vi "HAPS_LoadTable_Manual_Selected_Any_Preamp.vi"() -> ()   [LabVIEW 2023, in "HAPS.lvlib"]
uses:
  HAPS.lvlib
  set_ele.ctl
  HAPS_SerialPort.ctl
  HAPS_MCU_ELE_Func.ctl
  <vilib>/Utility/file.llb/Read Delimited Spreadsheet (string).vi
  R_S/R_S.lvlib
panel:
  in  "file path":path=path "D:/_Project/_Code/LabVIEW/_CLC_Gen4/CLC_LV2023/CLC_Cali/Log/HAPS/Preset.csv"
  in  "Preamp_Channel":bool[](array[boolean])
  in  "offset":i32=16
  in  "H_V?":bool
  in  "IC_On/OFF":bool[][](array[boolean])=[[FALSE, FALSE, FALSE, FALSE, FALSE, FALSE, FALSE, FALSE, FALSE, FALSE, FALSE, FALSE], [FALSE, FALSE, FALSE, FALSE, FALSE, FALSE, FALSE, FALSE, FALSE, FALSE, FALSE, FALSE], [FALSE, FALSE, FALSE, FALSE, FALSE, FALSE, FALSE, FALSE, FALSE, FALSE, FALSE, FALSE]]
  in  "ele_gain?":i32=35
  in  "sys reboot?":bool=TRUE
  in  "VISA resource name":refnum<visa-resource-name>="COM1"
  out "error IO":errorcluster
  out "Err_code":i32
  out "status":bool
  in  "offset?":bool
  in  "simu.?":bool
  in  "set_ele":T1={"ch"=0, "chain_id"=0, "group"=0, "array_id"=0, "ele_phase"=0, "ele_gain"=35, "com_gain"=17, "pd_range"=0}
  out "ele phase":i32
  out "ele gain":i32
  out "channel":i32
  out "chain ID":i32
  out "group":i32
  out "array id":i32
  # "HAPS 24x24 Setting Manual In-Phase : \n                                              Any BFIC & Preamp"
  # "Tx:35\nRx:22"
  # "0"
  # "5"
  # "6"
  # "11"
  # "Group_0"
  # "Group_1"
  # "Group_2"
  # "Not using!!!!!!!!!!!!!!!!!!!!!!!!!!!!!!!!!!!!!!!!"
  # "0        1       2        3        4       5        6       7        8        9      10      11     12     13     14      15"
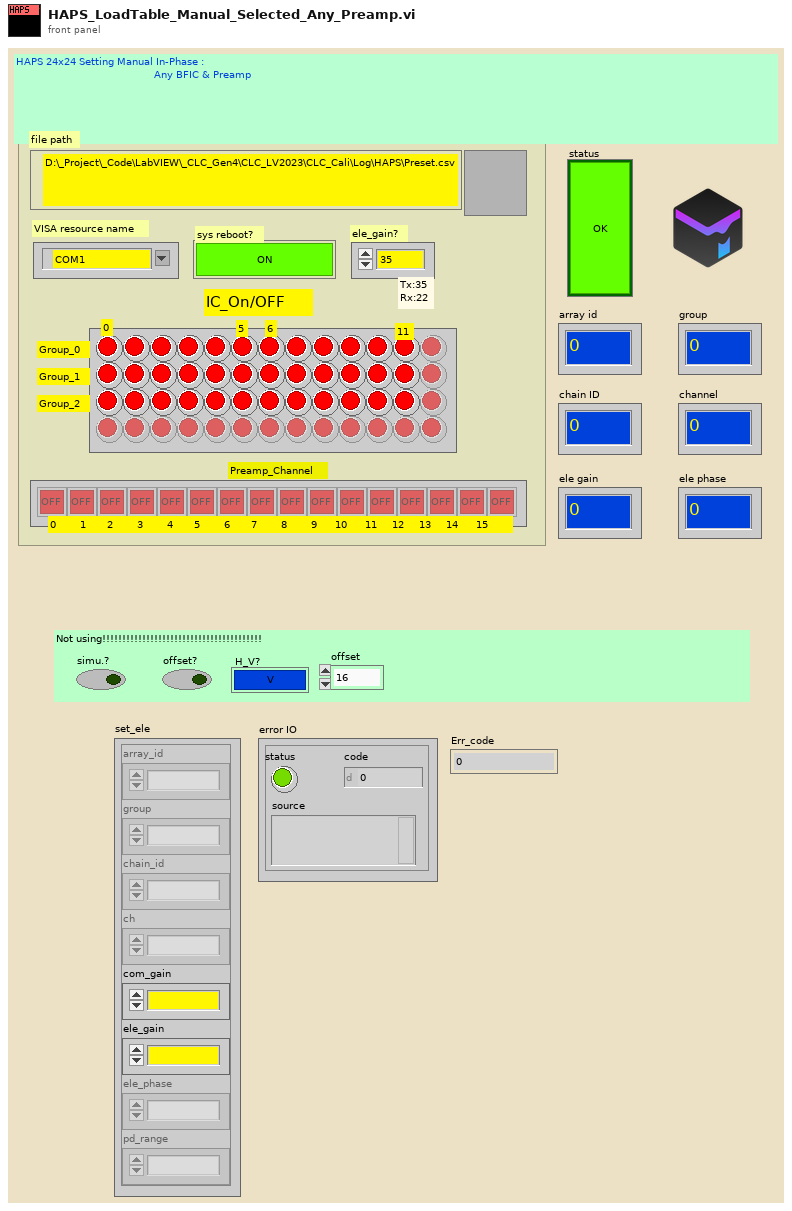
[diagram p1: front panel]
types:
  T1 = typedef "HAPS.lvlib/set_ele.ctl" = cluster{"ch":i32, "chain_id":i32, "group":i32, "array_id":i32, "ele_phase":i32, "ele_gain":i32, "com_gain":i32, "pd_range":i32}
  T2 = typedef "HAPS.lvlib/HAPS_SerialPort.ctl" = enum16{"Init", "Close", "CMD", "Flush"}
  T3 = typedef "HAPS.lvlib/HAPS_MCU_ELE_Func.ctl" = enum16{"array_init", "set_com_gain", "set_ch_gain_phase", "set_pd_range", "get_preamp_temp", "get_bfic_temp", "get_tx_pd", "ch_on", "ch_on_2", "ch_ctrl_all", "array_ctrl_src"}
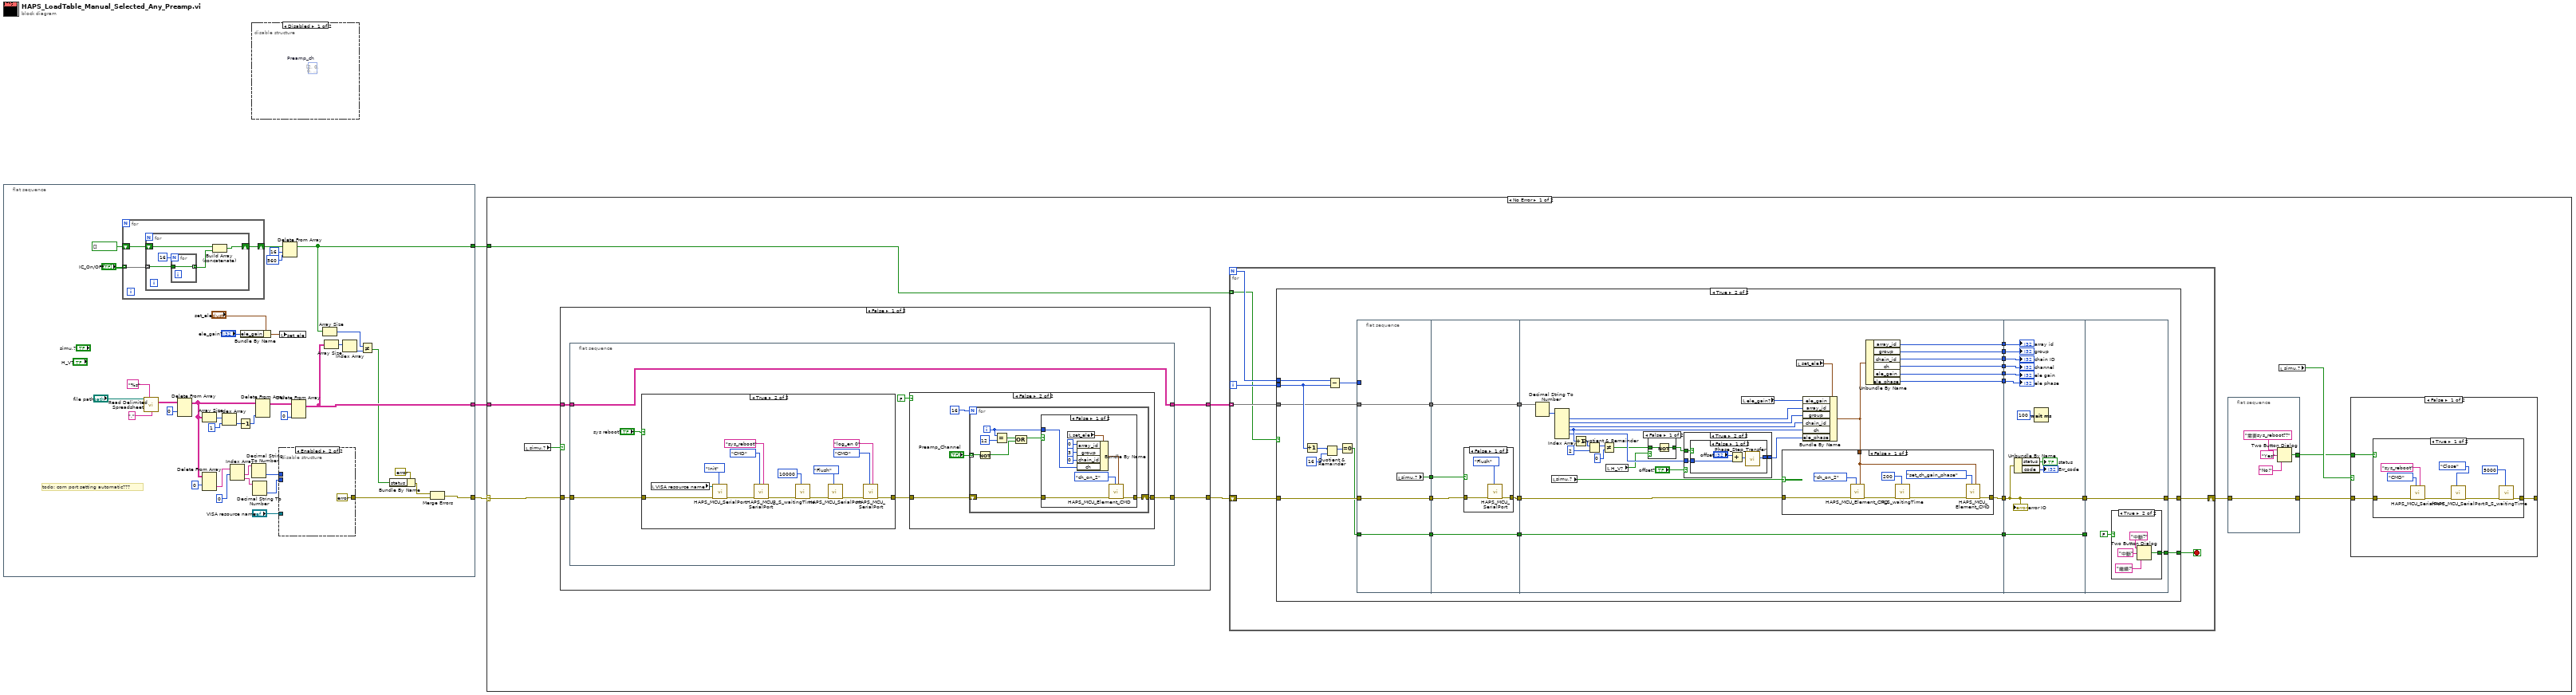
[diagram p0: block diagram]
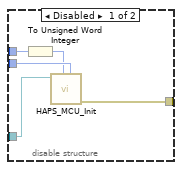
[diagram p2: hidden frame]
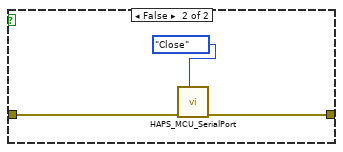
[diagram p4: hidden frame]
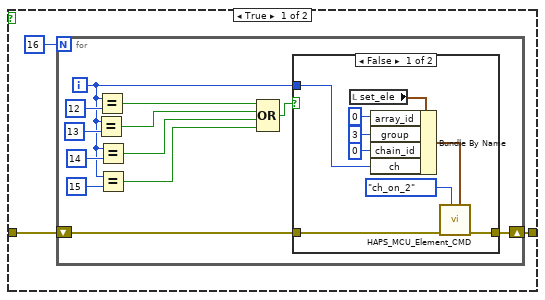
[diagram p6: hidden frame]
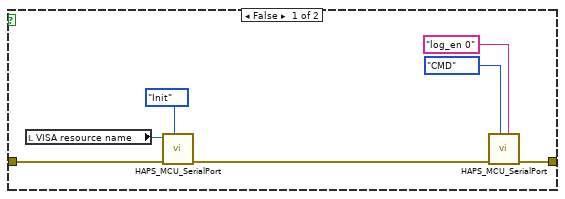
[diagram p9: hidden frame]
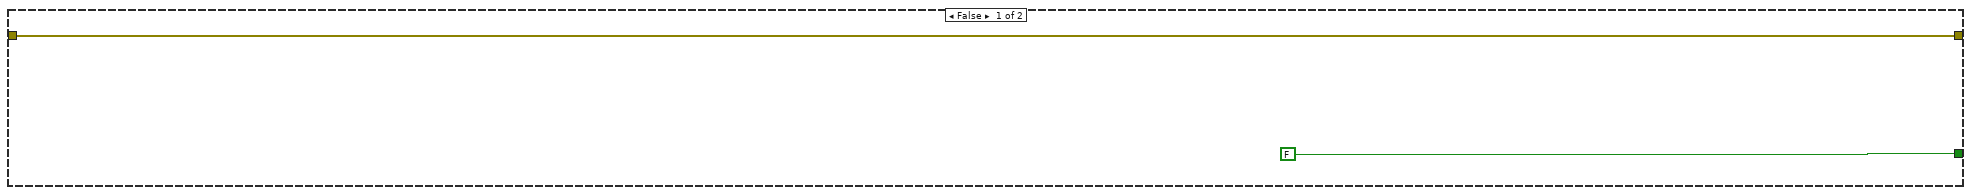
[diagram p11: hidden frame]
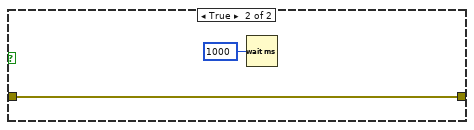
[diagram p16: hidden frame]
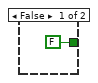
[diagram p17: hidden frame]
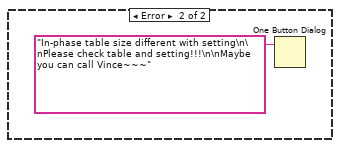
[diagram p18: hidden frame]
diagram:
  n1 = flat-sequence {
    tunnel: [w7] -> w3
    tunnel: [w11] -> w2
    tunnel: [w12] -> w1
    frame #0 {
      # "todo: com port setting automatic???"
      n2 = for {
        tunnel: "IC_On/OFF" -> [w44] mode=indexing
        shift-right: [w42] -> w17
        shift-left: bool[] [] -> [w43]
        n3 = for {
          tunnel: w44 -> [w48] mode=indexing
          shift-right: [w45] -> w42
          shift-left: w43 -> [w46]
          n4 = for {
            N: 16 -> [_]
            tunnel: w48 -> [w50]
            tunnel: [w50] -> w47 mode=indexing
          }
          n5 = Build Array (concatenate)(w46, w47) -> (w45:bool[])
        }
      }
      n6 = call-poly <vilib>:"Read Delimited Spreadsheet.vi"("file path (dialog if empty)"="file path", "format (%s)"="%s" ("format (%.3f)"), "delimiter (\\t)"="," ("delimiter (\\t)")) -> ("all rows"=w39:string[][])  [unwired: 7 in, 5 out]
      n7 = Delete From Array(array=w39, index (row)=0) -> (array with subset deleted=w29:string[][])  [unwired: 2 in, 1 out]
      n8 = Array Size(array=w29) -> (size(s)=w37:i32[])
      n9 = Delete From Array(array=w29, index (row)=0) -> (deleted portion=w28:string[])  [unwired: 2 in, 1 out]
      n10 = Index Array(array=w37, index=1) -> (element=w34:i32)
      n11 = Index Array(array=w28, index #1=0 ("index")) -> (element #1=w27:string, element #2=w26:string)  [unwired: 1 in]
      n12 = Decrement(x=w34) -> (x-1=w36:i32)
      n13 = Bundle By Name(cluster="set_ele", "ele_gain"="ele_gain?") -> (w18:T1)
      n14 = Decimal String To Number(string=w27) -> (number=w23:i32)  [unwired: 2 in, 1 out]
      n15 = Decimal String To Number(string=w26) -> (number=w22:i32)  [unwired: 2 in, 1 out]
      n16 = Delete From Array(array=w29, index (col)=w36) -> (array with subset deleted=w32:string[][])  [unwired: 2 in, 1 out]
      n17 = disable-structure shown="Enabled" {
        disable-tunnel: [w55 errorcluster {"status"=FALSE, "code"=0, "source"=""} ("error out")] -> w33
        disable-tunnel: w23 -> [w54 _]
        disable-tunnel: w22 -> [w53 _]
        disable-tunnel: "VISA resource name" -> [w52 _]
        frame Disabled {
          n18 = To Unsigned Word Integer(number=w54) -> (unsigned 16bit integer=w51:u16)
          n19 = call "HAPS_MCU_Init.vi"("array_id"=w53, "Tx/Rx"=w51, "VISA resource name"=w52) -> ("error out"=w55:errorcluster)  [unwired: 8 in]
        }
        frame Enabled {
        }
      }
      n20 = local write "set_ele"(w18) -> ()
      n21 = Delete From Array(array=w17, length=16, index=560) -> (array with subset deleted=w12:bool[])  [unwired: 1 out]
      n22 = Delete From Array(array=w32, index (col)=0 ("index (row)")) -> (array with subset deleted=w11:string[][])  [unwired: 2 in, 1 out]
      n23 = Array Size(array=w12) -> (size(s)=w9:i32)
      n24 = Array Size(array=w11) -> (size(s)=w10:i32[])
      n25 = Index Array(array=w10) -> (element=w8:i32)  [unwired: 1 in]
      n26 = Not Equal?(x=w9, y=w8) -> (x != y?=w5:bool)
      n27 = Bundle By Name(cluster=errorcluster {"status"=FALSE, "code"=0, "source"=""} ("error out"), "status"=w5) -> (w4:errorcluster)
      n28 = Merge Errors(w4, w33) -> (w7:errorcluster)
    }
  }
  n29 = disable-structure shown="Disabled" {
    frame Disabled {
      (unwired) i32[][] [[2, 0, 0, 8, 8, 10, 11, 9, 9, 1, 1, 3], [3, 1, 1, 9, 9, 11, 13, 15, 15, 7, 7, 5], [5, 7, 7, 15, 15, 13, 14, 14, 6, 6, 4, 12]]  # Preamp_ch
    }
    frame Enabled {
    }
  }
  n30 = case shown="No Error" w3 {
    selector: w3 -> [w64 _]
    tunnel: w2 -> [w66 _]
    tunnel: w1 -> [w60 _]
    frame No Error {
      n31 = local read "simu.?"() -> (w62:bool)
      n32 = case shown="False" w62 {
        tunnel: w66 -> [w90 w166]
        tunnel: [w89 w166] -> w65
        tunnel: w64 -> [w88 w165]
        tunnel: [w87 w165] -> w63
        frame False {
          n33 = flat-sequence {
            tunnel: w90 -> [w96]
            tunnel: [w96] -> w89
            tunnel: w88 -> [w94]
            tunnel: [w95] -> w87
            frame #0 {
              n34 = case shown="True" "sys reboot?" {
                tunnel: w94 -> [w148 w162]
                tunnel: [w146 w160] -> w93
                frame False {
                  n35 = local read "VISA resource name"() -> (w144:refnum<visa-resource-name>)
                  n36 = call "HAPS_MCU_SerialPort.vi"("HAPS_SerialPort_Func"=HAPS_SerialPort."Init", "error in"=w148, "VISA resource name"=w144) -> ("error out"=w145:errorcluster)  [unwired: 6 in, 2 out]
                  n37 = call "HAPS_MCU_SerialPort.vi"("Command"="log_en 0", "HAPS_SerialPort_Func"=enum16{"Init", "Close", "CMD"}."CMD" ("HAPS_SerialPort"), "error in"=w145) -> ("error out"=w146:errorcluster)  [unwired: 6 in, 2 out]
                }
                frame True {
                  n38 = local read "VISA resource name"() -> (w151:refnum<visa-resource-name>)
                  n39 = call "HAPS_MCU_SerialPort.vi"("HAPS_SerialPort_Func"=HAPS_SerialPort."Init", "error in"=w162, "VISA resource name"=w151) -> ("error out"=w157:errorcluster)  [unwired: 6 in, 2 out]
                  n40 = call "HAPS_MCU_SerialPort.vi"("Command"="sys_reboot", "HAPS_SerialPort_Func"=enum16{"Init", "Close", "CMD"}."CMD" ("HAPS_SerialPort"), "error in"=w157) -> ("error out"=w156:errorcluster)  [unwired: 6 in, 2 out]
                  n41 = call "R_S_waitingTime.vi"("Waiting Time(ms)"=u32 10000, "error in"=w156) -> ("error out"=w154:errorcluster)  [unwired: 9 in]
                  n42 = call "HAPS_MCU_SerialPort.vi"("HAPS_SerialPort_Func"=HAPS_SerialPort."Flush", "error in"=w154) -> ("error out"=w152:errorcluster)  [unwired: 7 in, 2 out]
                  n43 = call "HAPS_MCU_SerialPort.vi"("Command"="log_en 0", "HAPS_SerialPort_Func"=enum16{"Init", "Close", "CMD"}."CMD" ("HAPS_SerialPort"), "error in"=w152) -> ("error out"=w160:errorcluster)  [unwired: 6 in, 2 out]
                }
              }
              n44 = case shown="False" FALSE {
                tunnel: [w98 w124] -> w95
                tunnel: w93 -> [w97 w123]
                frame True {
                  n45 = for {
                    N: 16 -> [_]
                    shift-right: [w110] -> w98
                    shift-left: w97 -> [w111]
                    i -> [w101]
                    n46 = Equal?(x=w101, y=13) -> (x = y?=w105:bool)
                    n47 = Equal?(x=w101, y=12) -> (x = y?=w109:bool)
                    n48 = Equal?(x=w101, y=14) -> (x = y?=w103:bool)
                    n49 = Equal?(x=w101, y=15) -> (x = y?=w100:bool)
                    n50 = Compound Arithmetic op=OR(w109, w105, w103, w100) -> (w106:bool)
                    n51 = case shown="False" w106 {
                      tunnel: w111 -> [w114 w121]
                      tunnel: [w113 w121] -> w110
                      tunnel: w101 -> [w112 _]
                      frame False {
                        n52 = local read "set_ele"() -> (w116:T1)
                        n53 = Bundle By Name(cluster=w116, "array_id"=0, "group"=3, "chain_id"=0, "ch"=w112) -> (w117:T1)
                        n54 = call "HAPS_MCU_Element_CMD.vi"("set_ele"=w117, "HAPS_MCU_ELE_Func."=HAPS_MCU_ELE_Func."ch_on_2", "error in"=w114) -> ("error out"=w113:errorcluster)  [unwired: 7 in, 1 out]
                      }
                      frame True {
                      }
                    }
                  }
                }
                frame False {
                  n55 = for {
                    N: 16 -> [_]
                    shift-right: [w132] -> w124
                    shift-left: w123 -> [w133]
                    tunnel: "Preamp_Channel" -> [w127] mode=indexing
                    i -> [w130]
                    n56 = Not(x=w127) -> (.not. x?=w126:bool)
                    n57 = Equal?(x=w130, y=12) -> (x = y?=w129:bool)
                    n58 = Compound Arithmetic op=OR(w129, w126) -> (w128:bool)
                    n59 = case shown="False" w128 {
                      tunnel: w133 -> [w136 w143]
                      tunnel: [w135 w143] -> w132
                      tunnel: w130 -> [w134 _]
                      frame False {
                        n60 = local read "set_ele"() -> (w138:T1)
                        n61 = Bundle By Name(cluster=w138, "array_id"=0, "group"=3, "chain_id"=0, "ch"=w134) -> (w139:T1)
                        n62 = call "HAPS_MCU_Element_CMD.vi"("set_ele"=w139, "HAPS_MCU_ELE_Func."=HAPS_MCU_ELE_Func."ch_on_2", "error in"=w136) -> ("error out"=w135:errorcluster)  [unwired: 7 in, 1 out]
                      }
                      frame True {
                      }
                    }
                  }
                }
              }
            }
          }
        }
        frame True {
        }
      }
      n63 = for {
        N -> [w171]
        tunnel: w65 -> [w169] mode=indexing
        shift-right: [w173] -> w59
        shift-left: w63 -> [w172]
        tunnel: w60 -> [w167] mode=indexing
        i -> [w170]
        stop <- w168 stop-if-true
        n64 = case shown="True" w167 {
          tunnel: [w174 w187] -> w173
          tunnel: w172 -> [w174 w186]
          tunnel: w171 -> [_ w185]
          tunnel: w170 -> [_ w184]
          tunnel: w169 -> [_ w183]
          tunnel: [FALSE ("T button?") w177] -> w168
          frame False {
          }
          frame True {
            n65 = Increment(x=w184) -> (x+1=w181:i32)
            n66 = Quotient & Remainder(x=w181, y=16) -> (x-y*floor(x/y)=w179:i32)  [unwired: 1 out]
            n67 = Subtract(x=w185, y=w184) -> (x-y=w182:i32)
            n68 = Equal To 0?(x=w179) -> (x = 0?=w178:bool)
            n69 = flat-sequence {
              tunnel: w182 -> [_]
              tunnel: w186 -> [w206]
              tunnel: w183 -> [w207]
              tunnel: [w207] -> w203
              tunnel: [w206] -> w202
              tunnel: w178 -> [w205]
              tunnel: [w205] -> w201
              tunnel: [w204] -> w176
              tunnel: [w212] -> w200
              tunnel: [w211] -> w199
              tunnel: w203 -> [w212]
              tunnel: w202 -> [w210]
              tunnel: w201 -> [w209]
              tunnel: [w209] -> w198
              tunnel: w176 -> [w208]
              tunnel: w200 -> [w245]
              tunnel: w199 -> [w243]
              tunnel: [w231] -> w197
              tunnel: [w241] -> w196
              tunnel: [w240] -> w195
              tunnel: [w239] -> w194
              tunnel: [w238] -> w193
              tunnel: [w237] -> w192
              tunnel: [w236] -> w191
              tunnel: w198 -> [w232]
              tunnel: [w232] -> w190
              tunnel: w197 -> [w270]
              tunnel: w196 -> [w278]
              tunnel: w195 -> [w277]
              tunnel: w194 -> [w276]
              tunnel: w193 -> [w275]
              tunnel: w192 -> [w274]
              tunnel: w191 -> [w273]
              tunnel: [w270] -> w189
              tunnel: w190 -> [w271]
              tunnel: [w271] -> w188
              tunnel: w189 -> [w281]
              tunnel: w188 -> [_]
              tunnel: [w281] -> w187
              tunnel: [w280] -> w177
              frame #0 {
                n70 = local read "simu.?"() -> (w204:bool)
              }
              frame #1 {
                n71 = case shown="False" w208 {
                  tunnel: [w215 w216] -> w211
                  tunnel: w210 -> [w214 w216]
                  frame False {
                    n72 = call "HAPS_MCU_SerialPort.vi"("HAPS_SerialPort_Func"=HAPS_SerialPort."Flush", "error in"=w214) -> ("error out"=w215:errorcluster)  [unwired: 7 in, 2 out]
                  }
                  frame True {
                  }
                }
              }
              frame #2 {
                n73 = Decimal String To Number(string=w245) -> (number=w244:i32[])  [unwired: 2 in, 1 out]
                n74 = local read "simu.?"() -> (w230:bool)
                n75 = Index Array(array=w244) -> (element #1=w242:i32, element #2=w235:i32, element #3=w234:i32, element #4=w228:i32, element #5=w224:i32)  [unwired: 6 in, 1 out]
                n76 = Increment(x=w228) -> (x+1=w221:i32)
                n77 = Quotient & Remainder(x=w221, y=2) -> (x-y*floor(x/y)=w226:i32)  [unwired: 1 out]
                n78 = Not Equal?(x=w226, y=0) -> (x != y?=w218:bool)
                n79 = local read "H_V?"() -> (w219:bool)
                n80 = case shown="False" w219 {
                  tunnel: w218 -> [w247 w248]
                  tunnel: [w246 w248] -> w217
                  frame False {
                    n81 = Not(x=w247) -> (.not. x?=w246:bool)
                  }
                  frame True {
                  }
                }
                n82 = case shown="True" "offset?" {
                  tunnel: w224 -> [w249 w252]
                  tunnel: w217 -> [_ w251]
                  tunnel: [w249 w250] -> w223
                  frame False {
                  }
                  frame True {
                    n83 = case shown="False" w251 {
                      tunnel: w252 -> [w256 w257]
                      tunnel: [w253 w257] -> w250
                      frame False {
                        n84 = Add(x="offset", y=w256) -> (x+y=w254:i32)
                        n85 = call "Phase_Step_Transfer.vi"("Input_Phase_Step"=w254) -> ("Output_Phase_Step"=w253:i32)  [unwired: 10 in]
                      }
                      frame True {
                      }
                    }
                  }
                }
                n86 = local read "ele_gain?"() -> (w220:i32)
                n87 = local read "set_ele"() -> (w233:T1)
                n88 = Bundle By Name(cluster=w233, "ele_gain"=w220, "array_id"=w242, "group"=w235, "chain_id"=w234, "ch"=w228, "ele_phase"=w223) -> (w229:T1)
                n89 = case shown="False" w230 {
                  tunnel: w243 -> [w265 w267]
                  tunnel: w229 -> [w264 _]
                  tunnel: [w263 w267] -> w231
                  frame False {
                    n90 = call "HAPS_MCU_Element_CMD.vi"("set_ele"=w264, "HAPS_MCU_ELE_Func."=HAPS_MCU_ELE_Func."ch_on_2", "error in"=w265) -> ("error out"=w259:errorcluster)  [unwired: 7 in, 1 out]
                    n91 = call "R_S_waitingTime.vi"("Waiting Time(ms)"=u32 200, "error in"=w259) -> ("error out"=w258:errorcluster)  [unwired: 9 in]
                    n92 = call "HAPS_MCU_Element_CMD.vi"("set_ele"=w264, "HAPS_MCU_ELE_Func."=HAPS_MCU_ELE_Func."set_ch_gain_phase", "error in"=w258) -> ("error out"=w263:errorcluster)  [unwired: 7 in, 1 out]
                  }
                  frame True {
                    n93 = Wait (ms)(milliseconds to wait=u32 1000) -> ()  [unwired: 1 out]
                  }
                }
                n94 = Unbundle By Name(w229) -> ("array_id"=w241:i32, "group"=w240:i32, "chain_id"=w239:i32, "ch"=w238:i32, "ele_gain"=w237:i32, "ele_phase"=w236:i32)
              }
              frame #3 {
                n95 = Unbundle By Name(w270) -> ("status"=→"status":bool, "code"=→"Err_code":i32)
                n96 = Wait (ms)(milliseconds to wait=u32 100) -> ()  [unwired: 1 out]
                "group" <- w277
                "chain ID" <- w276
                "channel" <- w275
                "ele gain" <- w274
                "ele phase" <- w273
                "array id" <- w278
                "error IO" <- w270
              }
              frame #4 {
                n97 = case shown="True" FALSE {
                  tunnel: [FALSE ("T button?") w285] -> w280
                  frame False {
                  }
                  frame True {
                    n98 = Two Button Dialog(message="中斷?", 1:"繼續!" ("F button name (\"Cancel\")"), 2:"中斷" ("T button name (\"OK\")")) -> (T button?=w285:bool)
                  }
                }
              }
            }
          }
        }
      }
      n99 = flat-sequence {
        tunnel: w59 -> [w71]
        tunnel: [w71] -> w58
        tunnel: [w67] -> w57
        frame #0 {
          n100 = Two Button Dialog(message="需要sys_reboot??", 1:"No!" ("F button name (\"Cancel\")"), 2:"Yes" ("T button name (\"OK\")")) -> (T button?=w67:bool)
        }
      }
      n101 = local read "simu.?"() -> (w61:bool)
      n102 = case shown="False" w61 {
        tunnel: [w73 w86] -> _
        tunnel: w58 -> [w74 w86]
        tunnel: w57 -> [w72 _]
        frame False {
          n103 = case shown="True" w72 {
            tunnel: w74 -> [w82 w84]
            tunnel: [w75 w83] -> w73
            frame True {
              n104 = call "HAPS_MCU_SerialPort.vi"("Command"="sys_reboot", "HAPS_SerialPort_Func"=enum16{"Init", "Close", "CMD"}."CMD" ("HAPS_SerialPort"), "error in"=w82) -> ("error out"=w78:errorcluster)  [unwired: 6 in, 2 out]
              n105 = call "HAPS_MCU_SerialPort.vi"("HAPS_SerialPort_Func"=HAPS_SerialPort."Close", "error in"=w78) -> ("error out"=w76:errorcluster)  [unwired: 7 in, 2 out]
              n106 = call "R_S_waitingTime.vi"("Waiting Time(ms)"=u32 5000, "error in"=w76) -> ("error out"=w75:errorcluster)  [unwired: 9 in]
            }
            frame False {
              n107 = call "HAPS_MCU_SerialPort.vi"("HAPS_SerialPort_Func"=HAPS_SerialPort."Close", "error in"=w84) -> ("error out"=w83:errorcluster)  [unwired: 7 in, 2 out]
            }
          }
        }
        frame True {
        }
      }
    }
    frame Error {
      n108 = One Button Dialog(message="In-phase table size different with setting\n\nPlease check table and setting!!!\n\nMaybe you can call Vince~~~") -> ()  [unwired: 1 in, 1 out]
    }
  }
